vi "1.2.vi"(1 "n":dbl) -> (0 "f(n)":i32)   [LabVIEW 2013]
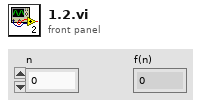
[diagram p1: front panel]
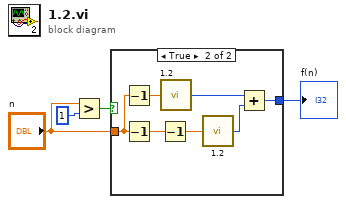
[diagram p0: block diagram]
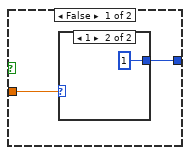
[diagram p2: hidden frame]
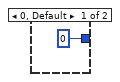
[diagram p3: hidden frame]
diagram:
  n1 = Greater?(x="n", y=1) -> (0:w3:bool)
  n2 = case shown="True" w3 {
    tunnel: "n" -> [w6 w14]
    tunnel: [w5 w9] -> w1
    frame False {
      n3 = case shown="1" w6 {
        tunnel: [0 1] -> w5
        frame 0, Default {
        }
        frame 1 {
        }
      }
    }
    frame True {
      n4 = Decrement(x=w14) -> (x-1=w15:dbl)
      n5 = Decrement(x=w14) -> (x-1=w13:dbl)
      n6 = Decrement(x=w13) -> (x-1=w12:dbl)
      n7 = call "1.2.vi"("n"=w15) -> ("f(n)"=w11:i32)
      n8 = call "1.2.vi"("n"=w12) -> ("f(n)"=w10:i32)
      n9 = Add(x=w11, y=w10) -> (x+y=w9:i32)
    }
  }
  "f(n)" <- w1
